vi "Mask_Color.vi"(0 "Image_3d":u8[][][](array[numeric]), 5 "error in (no error)":errorcluster, 7 "ColorMask Low/High":u8[][](array[numeric])=[[0, 100], [200, 255], [170, 230]]) -> (12 "ticks (ms)":u32, 14 "Image_2d":i16[][](array[numeric]), 19 "error out":errorcluster)   [LabVIEW 2016]
panel:
  out "Intensity Graph":i16[][](graph)
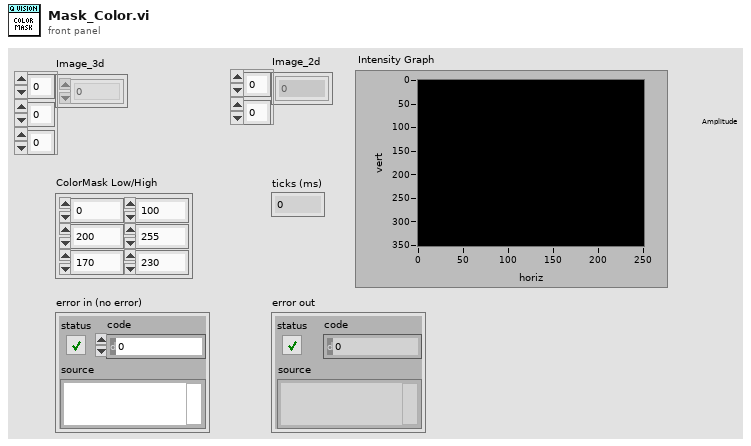
[diagram p1: front panel]
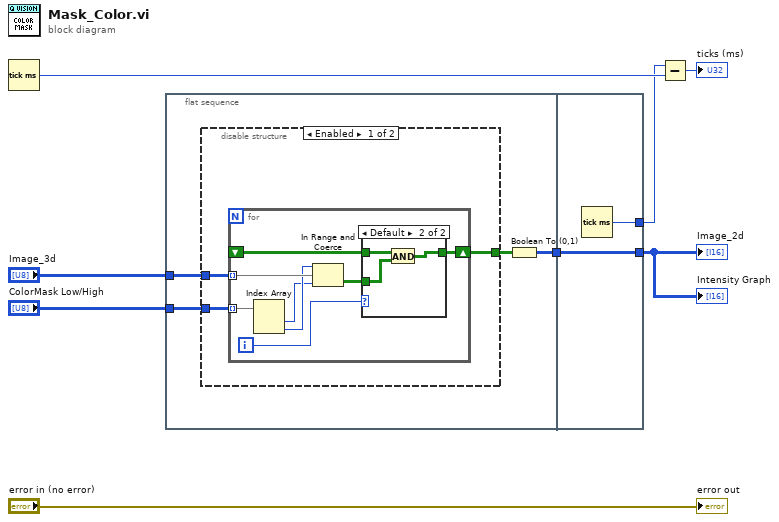
[diagram p0: block diagram]
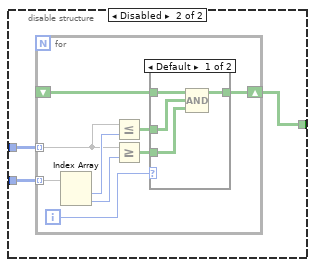
[diagram p3: hidden frame]
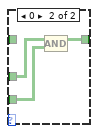
[diagram p4: hidden frame]
diagram:
  n1 = Tick Count (ms)() -> (millisecond timer value=w4:u32)
  n2 = flat-sequence {
    tunnel: "Image_3d" -> [w12]
    tunnel: "ColorMask Low/High" -> [w11]
    tunnel: [w9] -> w2
    tunnel: [w48] -> w5
    tunnel: w2 -> [w48]
    tunnel: [w47] -> w1
    frame #0 {
      n3 = disable-structure shown="Enabled" {
        disable-tunnel: w12 -> [w15 w30]
        disable-tunnel: w11 -> [w14 w29]
        disable-tunnel: [w13 w28] -> w10
        frame Enabled {
          n4 = for {
            tunnel: w15 -> [w23] mode=indexing
            tunnel: w14 -> [w22] mode=indexing
            shift-right: [w20] -> w13
            shift-left: _ -> [w19]
            i -> [w21]
            n5 = Index Array(array=w22) -> (element #1=w16:u8, element #2=w17:u8)  [unwired: 2 in]
            n6 = In Range and Coerce(upper limit=w17, x=w23, lower limit=w16) -> (In Range?=w18:bool[][])  [unwired: 1 out]
            n7 = case shown="Default" w21 {
              tunnel: [w24 w25] -> w20
              tunnel: w18 -> [w24 w26]
              tunnel: w19 -> [_ w27]
              frame 0 {
              }
              frame Default {
                n8 = And(x=w27, y=w26) -> (x .and. y?=w25:bool[][])
              }
            }
          }
        }
        frame Disabled {
          n9 = for {
            tunnel: w30 -> [w34] mode=indexing
            tunnel: w29 -> [w39] mode=indexing
            shift-right: [w37] -> w28
            shift-left: _ -> [w36]
            i -> [w38]
            n10 = Index Array(array=w39) -> (element #1=w35:u8, element #2=w33:u8)  [unwired: 2 in]
            n11 = Less Or Equal?(x=w34, y=w35) -> (x <= y?=w32:bool[][])
            n12 = Greater Or Equal?(x=w34, y=w33) -> (x >= y?=w31:bool[][])
            n13 = case shown="Default" w38 {
              tunnel: [w41 w45] -> w37
              tunnel: w32 -> [w42 w46]
              tunnel: w36 -> [w43 _]
              tunnel: w31 -> [w40 w44]
              frame Default {
                n14 = Compound Arithmetic op=AND(w43, w42, w40) -> (w41:bool[][])
              }
              frame 0 {
                n15 = Compound Arithmetic op=AND(w46, w44) -> (w45:bool[][])
              }
            }
          }
        }
      }
      n16 = Boolean To (0,1)(Boolean=w10) -> (0, 1=w9:i16[][])
    }
    frame #1 {
      n17 = Tick Count (ms)() -> (millisecond timer value=w47:u32)
    }
  }
  n18 = Subtract(x=w1, y=w4) -> (x-y=→"ticks (ms)":u32)
  "Image_2d" <- w5
  "error out" <- "error in (no error)"
  "Intensity Graph" <- w5
